vi "2nd_order_Poly_convert.vi"(3 "Calib constants":dbl[](array[numeric])=[0.2727, 22.328, 22.281, -22.056, 13.889] format="%.3e", 6 "Voltage":dbl[](array[numeric])) -> (1 "Eng Values":dbl[](array[numeric]))   [LabVIEW 2010]
panel:
  # "x^0\nx^1\nx^2\nx^3\nx^4"
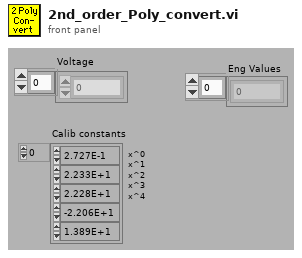
[diagram p1: front panel]
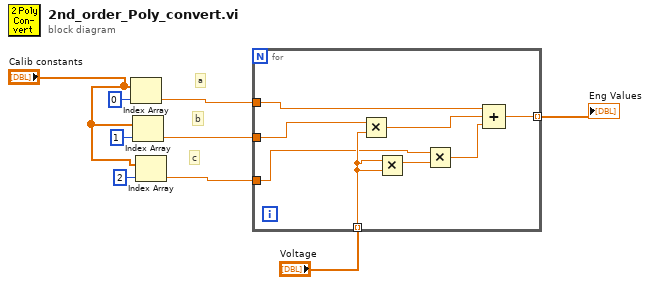
[diagram p0: block diagram]
diagram:
  # "c"
  # "b"
  # "a"
  n1 = Index Array(array="Calib constants", index=0) -> (element=w5:dbl)
  n2 = Index Array(array="Calib constants", index=1) -> (element=w4:dbl)
  n3 = Index Array(array="Calib constants", index=2) -> (element=w2:dbl)
  n4 = for {
    tunnel: w5 -> [w17]
    tunnel: w4 -> [w16]
    tunnel: "Voltage" -> [w14] mode=indexing
    tunnel: w2 -> [w12]
    tunnel: [w10] -> w1 mode=indexing
    n5 = Multiply(x=w16, y=w14) -> (x*y=w15:dbl)
    n6 = Multiply(x=w14, y=w14) -> (x*y=w13:dbl)
    n7 = Multiply(x=w12, y=w13) -> (x*y=w11:dbl)
    n8 = Compound Arithmetic op=ADD(w17, w15, w11) -> (w10:dbl)
  }
  "Eng Values" <- w1
